vi "RTTestApp.vi"() -> ()   [LabVIEW 2019]
uses:
  <vilib>/FPGAPlugInAG/roboRIO/niLvFpga_Open_roboRIO.vi
  <vilib>/rvi/interface/common/dynamic/niFpgaDynamicAddResources.vi
  <vilib>/Utility/error.llb/Error Cluster From Error Code.vi
  <vilib>/rvi/errors/niLvFpgaAdjustHostInterfaceError.vi
  <vilib>/rvi/interface/nirviOpenFPGA/nirviOpenFPGA.xnode
  FPGA Bitfiles/roboriofpga_OpenSourceRIO_OpenSourceRIO.lvbitx
  OpenSourceRIO.vi
  <vilib>/rvi/interface/nirviReadWriteControl/nirviReadWriteControl.xnode
  NiFpgaLv.dll
  <vilib>/rvi/interface/Simulation/niFpgaSimulationCallBeginRW.vi
panel:
  in  "PWM_FeedWatchdog":bool
  in  "PWM_MinHigh":u16
  in  "PWM_Period":u16
  in  "PWM_Squelch":u8[](array[numeric])=[0, 0, 0, 0, 0, 0, 0, 0, 0, 0]
  in  "PWM_0":u16
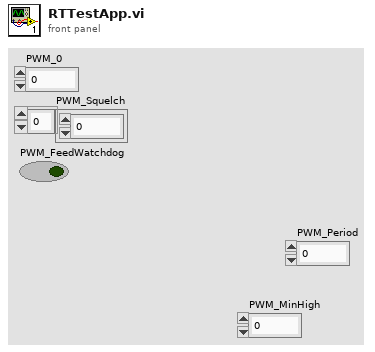
[diagram p1: front panel]
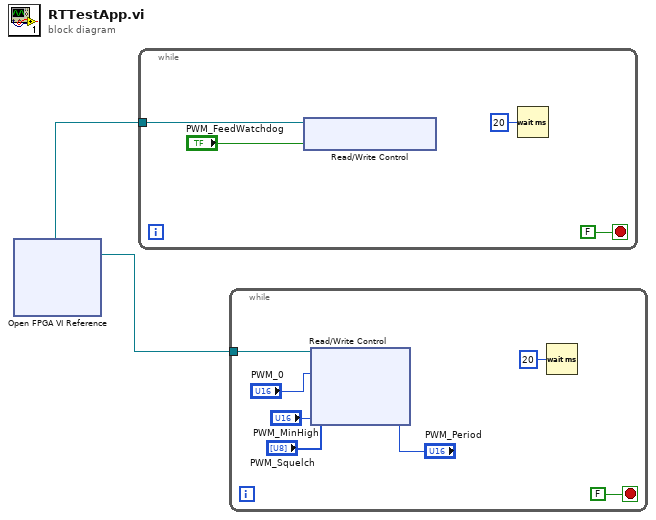
[diagram p0: block diagram]
diagram:
  n1 = xnode "Open FPGA VI Reference"() -> ("FPGA VI Reference Out"=w1:refnum<k20>)  [unwired: 2 in, 1 out]
  n2 = while {
    tunnel: w1 -> [w4]
    stop <- FALSE stop-if-true
    n3 = xnode "Read/Write Control"("FPGA VI Reference In"=w4, "PWM_FeedWatchdog"="PWM_FeedWatchdog") -> ()  [unwired: 1 in, 2 out]
    n4 = Wait (ms)(milliseconds to wait=u32 20) -> ()  [unwired: 1 out]
  }
  n5 = while {
    tunnel: w1 -> [w11]
    stop <- FALSE stop-if-true
    n6 = xnode "Read/Write Control"("FPGA VI Reference In"=w11, "PWM_0"="PWM_0", "PWM_Squelch"="PWM_Squelch", "PWM_Period"="PWM_Period", "PWM_MinHigh"="PWM_MinHigh") -> ()  [unwired: 1 in, 2 out]
    n7 = Wait (ms)(milliseconds to wait=u32 20) -> ()  [unwired: 1 out]
  }
